vi "FindEqualNameInComboBox(SubVI).vi"(8 "Error In":errorcluster, 10 "Name":string, 11 "Strings And Values[]":cluster{"String":string, "Value":string}[](array[cluster])) -> (0 "Error Out":errorcluster, 2 "NumPlot":dbl, 3 "Does the array contain this name?":bool)   [LabVIEW 2018]
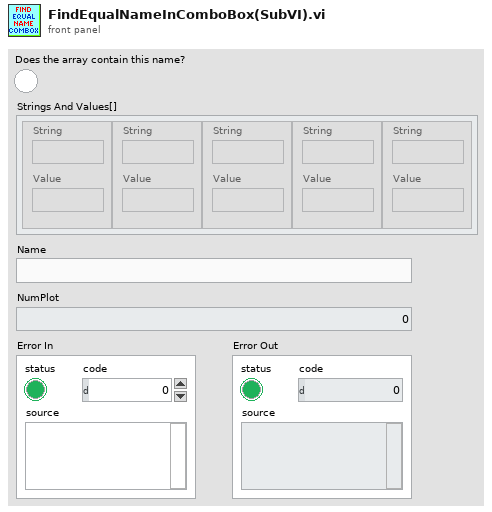
[diagram p1: front panel]
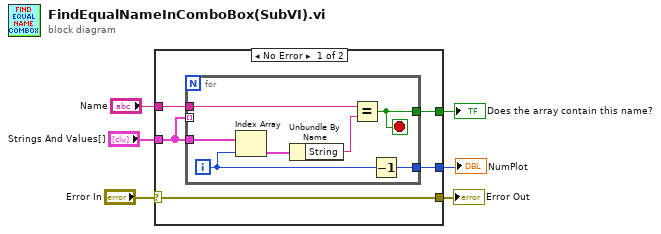
[diagram p0: block diagram]
diagram:
  n1 = case shown="No Error" "Error In" {
    selector: "Error In" -> [w7 w19]
    tunnel: [w11 _] -> w5
    tunnel: [w10 _] -> w4
    tunnel: "Strings And Values[]" -> [w9 _]
    tunnel: "Name" -> [w8 _]
    tunnel: [w7 w19] -> w1
    frame No Error {
      n2 = for {
        tunnel: w9 -> [_] mode=indexing
        tunnel: w9 -> [w18]
        tunnel: w8 -> [w16]
        tunnel: [w14] -> w11
        tunnel: [w13] -> w10
        i -> [w12]
        stop <- w14 stop-if-true
        n3 = Index Array(array=w18, index=w12) -> (element=w17:cluster{"String":string, "Value":string})
        n4 = Unbundle By Name(w17) -> ("String"=w15:string)
        n5 = Equal?(x=w16, y=w15) -> (x = y?=w14:bool)
        n6 = Decrement(x=w12) -> (x-1=w13:i32)
      }
    }
    frame Error {
    }
  }
  "Error Out" <- w1
  "Does the array contain this name?" <- w5
  "NumPlot" <- w4
